vi "updateEndTime.vi"(8 "error in (no error)":errorcluster, 11 "SingleToneRamp in":refnum<class "SingleToneRamp.lvclass">) -> (0 "error out":errorcluster, 3 "SingleToneRamp out":refnum<class "SingleToneRamp.lvclass">)   [LabVIEW 2009, in "Tools.lvlib" / "Scripting.lvlib" / "SingleToneRamp.lvclass"]
uses:
  SingleToneRamp.lvclass
  SingleToneRamp.lvclass/SingleToneRamp.ctl
  ScriptEvent.lvclass
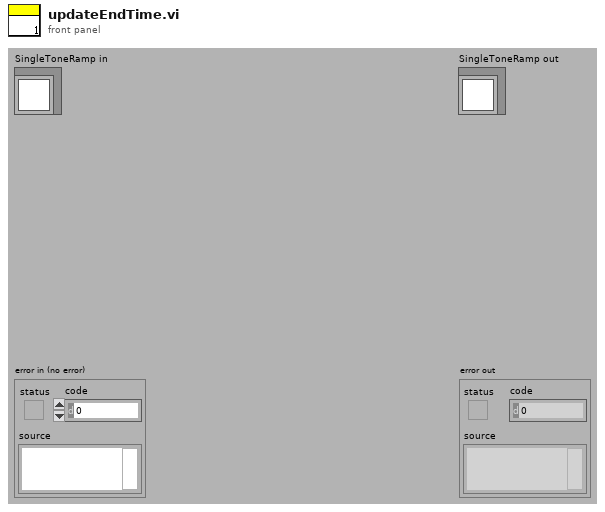
[diagram p1: front panel]
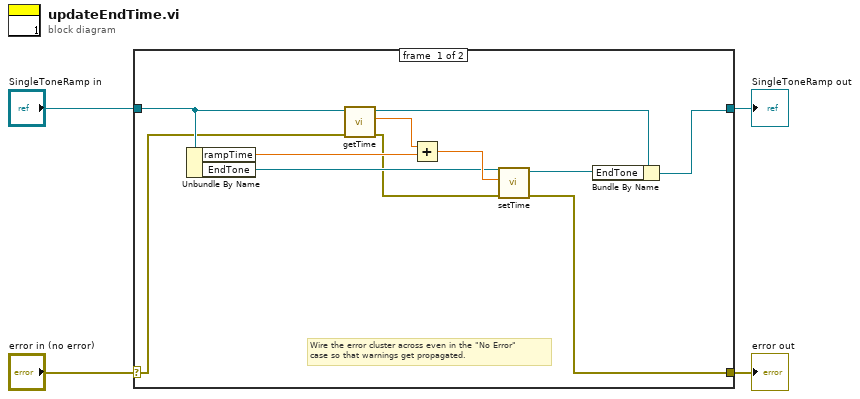
[diagram p0: block diagram]
diagram:
  n1 = case shown="No Error" "error in (no error)" {
    selector: "error in (no error)" -> [w5 w17]
    tunnel: [w7 w17] -> w3
    tunnel: [w8 w16] -> w1
    tunnel: "SingleToneRamp in" -> [w15 w16]
    frame #0 {
      # "Wire the error cluster across even in the \"No Error\"\ncase so that warnings get propagated."
      n2 = Unbundle By Name(w15) -> ("rampTime"=w13:dbl, "EndTone"=w11:refnum<class "SingleTone.lvclass">)
      n3 = call "getTime.vi"("error in (no error)"=w5, "ScriptEvent.lvclass in"=w15) -> ("error out"=w6:errorcluster, "time"=w14:dbl, "ScriptEvent.lvclass out"=w9:refnum<class "SingleToneRamp.lvclass">)  [unwired: 7 in]
      n4 = Add(x=w14, y=w13) -> (x+y=w12:dbl)
      n5 = call "setTime.vi"("error in (no error)"=w6, "time"=w12, "ScriptEvent.lvclass in"=w11) -> ("error out"=w7:errorcluster, "ScriptEvent.lvclass out"=w10:refnum<class "SingleTone.lvclass">)  [unwired: 7 in]
      n6 = Bundle By Name(cluster=w9, "EndTone"=w10) -> (w8:refnum<class "SingleToneRamp.lvclass">)
    }
    frame #1 {
    }
  }
  "error out" <- w3
  "SingleToneRamp out" <- w1
